vi "CANFD Get CAN Speed Arg.vi"(7 "SpeedBpsDBT":u32, 9 "SpeedBpsNBT":u32, 10 "pCanConfig":T1, 11 "DevHandle":i32) -> (2 "pCanConfig out":T1, 3 "function return":i32)   [LabVIEW 2010, in "usb2canfd.lvlib"]
doc: "int WINAPI CANFD_GetCANSpeedArg(int DevHandle, CANFD_INIT_CONFIG* pCanConfig, unsigned int SpeedBpsNBT, unsigned int SpeedBpsDBT);"
uses:
  usb2canfd.lvlib
  USB2XXX/trunk/USB2XXX/USB2XXX/vs2019/Release/USB2XXX.dll
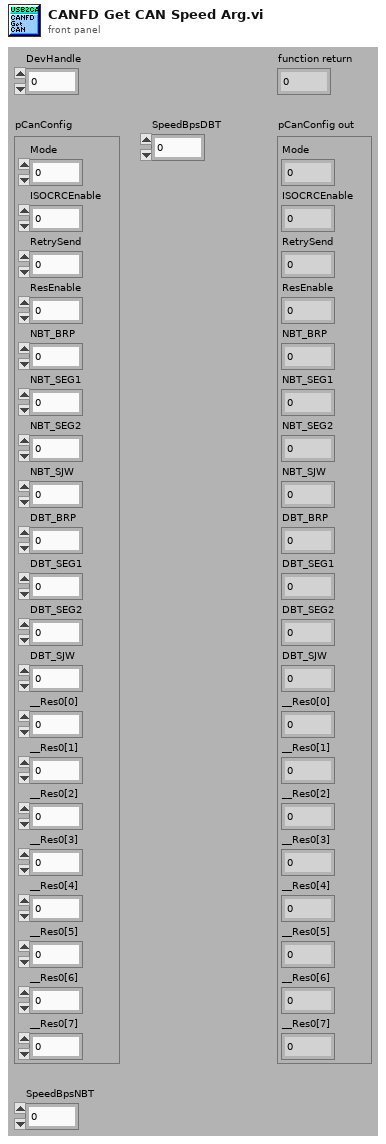
[diagram p1: front panel]
types:
  T1 = cluster{"Mode":u8, "ISOCRCEnable":u8, "RetrySend":u8, "ResEnable":u8, "NBT_BRP":u8, "NBT_SEG1":u8, "NBT_SEG2":u8, "NBT_SJW":u8, "DBT_BRP":u8, "DBT_SEG1":u8, "DBT_SEG2":u8, "DBT_SJW":u8, "__Res0[0]":u8, "__Res0[1]":u8, "__Res0[2]":u8, "__Res0[3]":u8, "__Res0[4]":u8, "__Res0[5]":u8, "__Res0[6]":u8, "__Res0[7]":u8}
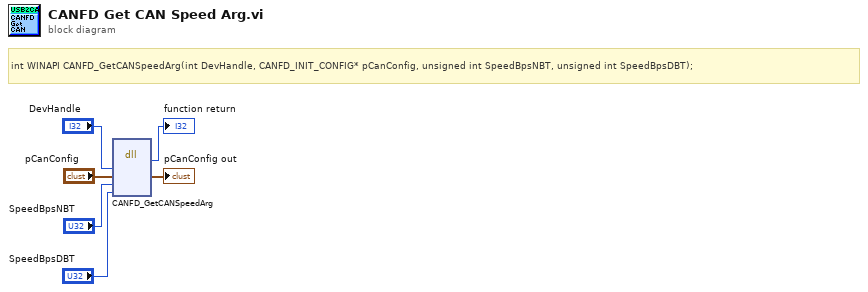
[diagram p0: block diagram]
diagram:
  # "int WINAPI CANFD_GetCANSpeedArg(int DevHandle, CANFD_INIT_CONFIG* pCanConfig, unsigned int SpeedBpsNBT, unsigned int SpeedBpsDBT);"
  n1 = dll-call lib="E:/Projects/USB2XXX/trunk/USB2XXX/USB2XXX/vs2019/Release/USB2XXX.*" fn="CANFD_GetCANSpeedArg"("DevHandle"="DevHandle", "pCanConfig"="pCanConfig", "SpeedBpsNBT"="SpeedBpsNBT", "SpeedBpsDBT"="SpeedBpsDBT") -> (→"function return":i32, "pCanConfig"=→"pCanConfig out":T1)  [unwired: 6 in, 2 out]
